vi "Constants.vi"() -> ()   [LabVIEW 2020, in "PXI-2514 Shared.lvlib"]
doc: "Use this Global VI to access the GUIDs assigned to the page resources of the Custom Device."
uses:
  PXI-2514 Shared.lvlib
panel:
  in  "Tab Control":enum32{"GUIDs", "Constants", "Properties"}(tab)
  in  "Disable PXI-2514 GUID":string="6368a457-2b09-4e67-8852-5a75b77cd864"
  in  "PXI-2514 Channel Page":string="73d9ba6a-5ac3-4ef9-bef9-f6783ddd9c22"
  in  "PXI-2514":string="874a7ebe-89ae-45e1-91d0-671ffa7b4cc5"
  in  "Channel Fault":string="Channel Fault"
  in  "FIU Channel #":string="FIU Channel #"
  in  "Hardware Device Name":string="Hardware Device Name"
  in  "Fault Channel Description":string="The \"Name (Alias)\" for each channel may be changed. The \"Hardware Channel #\" cannot be changed by the user, and represents the actual Fault Channel being controller.\n\nThe Fault Default Value sets the default state for the channel."
  in  "FIU Description":string="This is a Custom Device for the PXI-2514 FIU."
  in  "Compiled.Settings":string="Compiled.Settings"
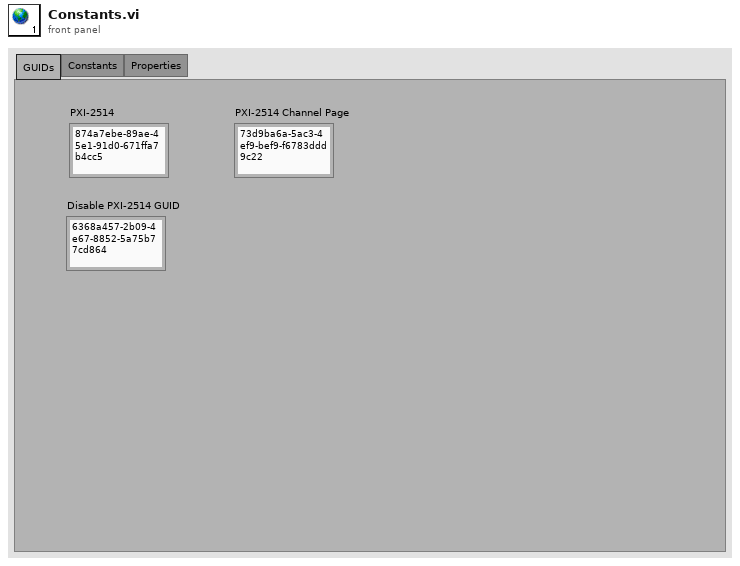
[diagram p1: front panel]
diagram:
